vi "speed debug.vi"() -> ()   [LabVIEW 2019]
uses:
  <vilib>/eio/EIONode/EIONode.xnode
  <vilib>/rvi/Analysis/measure/period/XNode/niFpgaAnalogPeriod.xnode
  <vilib>/rvi/Analysis/measure/period/templates/niFPGA Period Edge Direction.ctl
  <vilib>/rvi/eio/common/nirviEmuTemplateMethod_errors.vi
  <vilib>/rvi/Analysis/common/codeGenErrors/XNode/niFpgaXNodeCodeGenErrorHandle.vi
  <vilib>/Platform/TimedLoop/XDataNode/wakeup.ctl
  <vilib>/Platform/TimedLoop/XDataNode/XDNodeRunTimeDep.lvlib
  <vilib>/Platform/TimedLoop/XDataNode/nitl_modes.ctl
  <vilib>/Platform/TimedLoop/XDataNode/timing_clust.ctl
  <vilib>/Platform/TimedLoop/XDataNode/XDataNode.xnode
  <vilib>/rvi/Analysis/utilities/niFPGA Threshold Crossing Logic.vi
  <vilib>/rvi/Analysis/measure/dc-rms/XNode/niFpgaDC-RMS.xnode
  <vilib>/rvi/FXPMathLib/basic elements/FxpIntAccumulator/subVIs/nifxpmath_IntAccumulator_SimConfig.ctl
  <vilib>/rvi/FXPMathLib/basic elements/FxpIntAccumulator/simVIs/DllFxpIntAccumulator_sub.vi
  <vilib>/rvi/FXPMathLib/basic elements/FxpIntAccumulator/XNode/nifxpmath_IntAccumulator.xnode
  <vilib>/rvi/FXPMathLib/FxpMul/XNode/nifxpmath_Multiplier.xnode
  <vilib>/rvi/FXPMathLib/sim/FxpSim.dll
  <vilib>/rvi/Analysis/measure/mean-var-std/XNode/niFpgaMean-Var-Std.xnode
  <vilib>/fxp/LVFixedPointOverflowPolicyTypeDef.ctl
  <vilib>/rvi/FXPMathLib/FxpSqrt/subVIs/nifxpmath_Sqrt_SimConfig.ctl
  <vilib>/rvi/FXPMathLib/FxpSqrt/simVIs/DllSqrtTemp_sub.vi
  <vilib>/rvi/FXPMathLib/FxpSqrt/XNode/nifxpmath_Sqrt.xnode
  <vilib>/rvi/FXPMathLib/FxpDiv/XNode/nifxpmath_Div.xnode
  <vilib>/rvi/FXPMathLib/FxpDiv/simVIs/DllFxpDivTemp_sub.vi
  <vilib>/rvi/FXPMathLib/FxpDiv/subVIs/nifxpmath_Div_SimConfig.ctl
  <vilib>/rvi/FXPMathLib/FxpAdd/XNode/nifxpmath_Add.xnode
panel:
  out "Mean Speed":fxp<+/-,32,19> format="%#.0f"
  out "Speed":fxp<+,32,18> format="%#.0f"
  out "RMS":fxp<+,24,6> format="%.1f"
  out "Current":fxp<+/-,24,6>
  out "AI0":fxp<+/-,24,5>
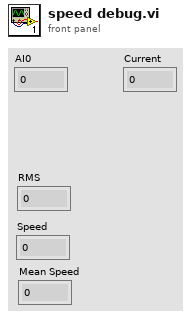
[diagram p1: front panel]
types:
  T1 = typedef "XDNodeRunTimeDep.lvlib/timing_clust.ctl" = cluster{"Expected End [f-1]":u64, "Actual End [f-1]":u64, "Finished Late? [f-1]":bool, "Expected End [i-1]":u64, "Actual End [i-1]":u64, "Finished Late? [i-1]":bool, "Expected Start [i]":u64, "Actual Start [i]":u64, "Expected Start [f]":u64, "Actual Start [f]":u64, "Source Name":string, "Structure Name":string, "Period":i64, "Deadline":i64, "Offset":i64, "Start":i64, "Priority":i32, "Timeout":i32, "Mode":T2, "Wakeup Reason":T3, "Error":errorcluster, "Source Type":string, "Secondary Source Type":string, "Global End Time":u64, "Global Start Time":u64, "Frame Duration":u64, "Iteration Duration":u64, "Assigned CPU":i32, "I/O Scan Engine Mode":u32}
  T2 = typedef "XDNodeRunTimeDep.lvlib/nitl_modes.ctl" = enum32{"No Change", "Process missed periods, maintain original phase", "Discard missed periods, maintain original phase", "Process missed periods, ignore original phase", "Discard missed periods, ignore original phase"}
  T3 = typedef "XDNodeRunTimeDep.lvlib/wakeup.ctl" = enum32{"Normal", "Aborted", "Asynchronous wakeup", "Timing source error", "Timed loop error", "Timeout"}
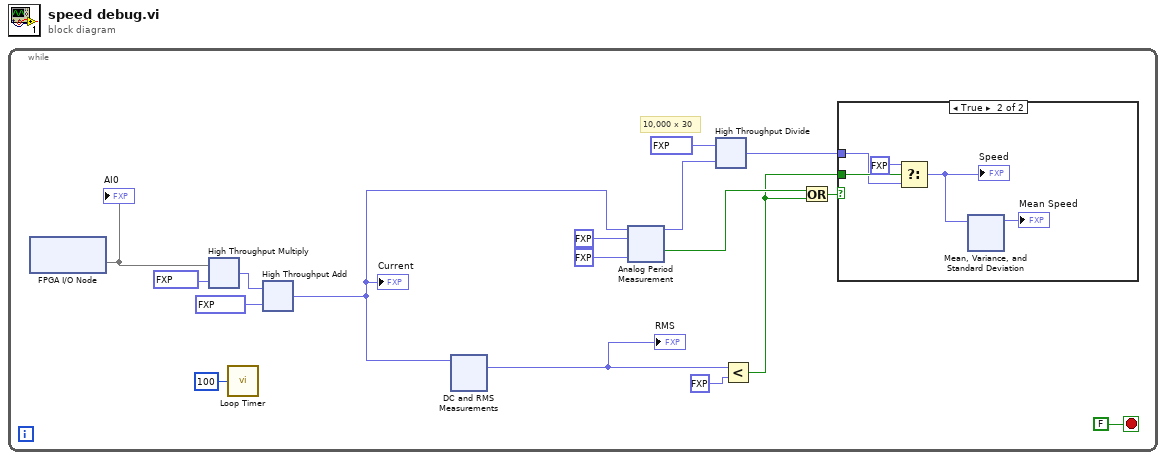
[diagram p0: block diagram]
diagram:
  n1 = while {
    stop <- FALSE stop-if-true
    # "10,000 x 30"
    n2 = xnode "FPGA I/O Node"() -> ("AI0"=w5)  [unwired: 1 in, 1 out]
    "AI0" <- w5
    n3 = xnode ("High Throughput Multiply")("x"=w5, "y"=fxp<+,16,5> 24.0380859375) -> ("x*y"=w3:fxp<+/-,40,10>)
    n4 = call "Loop Timer"("Count(uSec)"=u32 100) -> ()  [unwired: 1 out]
    n5 = xnode ("High Throughput Add")("x"=w3, "y"=fxp<+/-,18,7> -60.09521484375) -> ("x+y"=w1:fxp<+/-,24,6>)
    "Current" <- w1
    n6 = xnode ("DC and RMS Measurements")("input data"=w1) -> ("RMS"=w10:fxp<+,24,6>)  [unwired: 1 in, 1 out]
    "RMS" <- w10
    n7 = xnode ("Analog Period Measurement")("input data"=w1, "threshold level"=fxp<+/-,24,6> 0.0, "hysteresis"=fxp<+,23,5> 1.0) -> ("period (samples)"=w7:fxp<+,32,16>, "output valid"=w13:bool)  [unwired: 2 in, 2 out]
    n8 = xnode "High Throughput Divide"("x"=fxp<+,32,19> 300000.0, "y"=w7) -> ("x/y"=w6:fxp<+,32,18>)
    n9 = Less?(x=w10, y=fxp<+,24,6> 1.0 ("current threshold")) -> (x < y?=w11:bool)
    n10 = Or(x=w13, y=w11) -> (x .or. y?=w12:bool)
    n11 = case shown="True" w12 {
      tunnel: w6 -> [_ w156]
      tunnel: w11 -> [_ w157]
      frame False {
      }
      frame True {
        n12 = Select(t=fxp<+,32,18> 0.0 ("input data"), s=w157, f=w156) -> (s? t:f=w154:fxp<+,32,18>)
        "Speed" <- w154
        n13 = xnode ("Mean, Variance, and Standard Deviation")("input data"=w154) -> ("mean"=→"Mean Speed":fxp<+/-,32,19>)  [unwired: 1 in, 1 out]
      }
    }
  }
